vi "Regex Submatch Array.vi"(5 "multiline? (F)":bool, 6 "Submatches? (T)":bool=TRUE, 7 "ignore case? (F)":bool, 8 "error in (no error)":errorcluster, 9 "offset (0)":i32, 10 "regular expression":string, 11 "string":string) -> (0 "error out":errorcluster, 1 "offset past match":i32, 2 "after match":string, 3 "before match":string, 4 "matches":string[](array[string]))   [LabVIEW 2020, in "URI.lvlib"]
uses:
  URI.lvlib
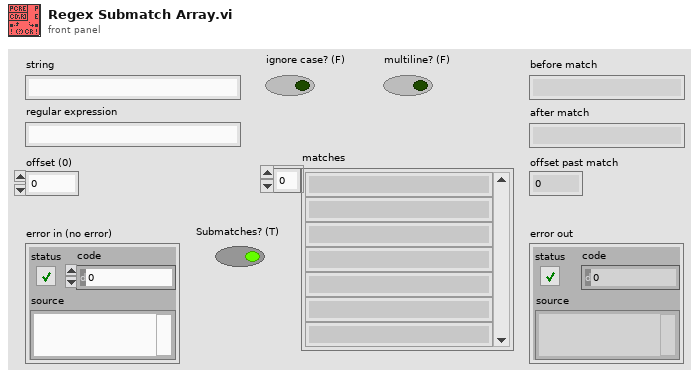
[diagram p1: front panel]
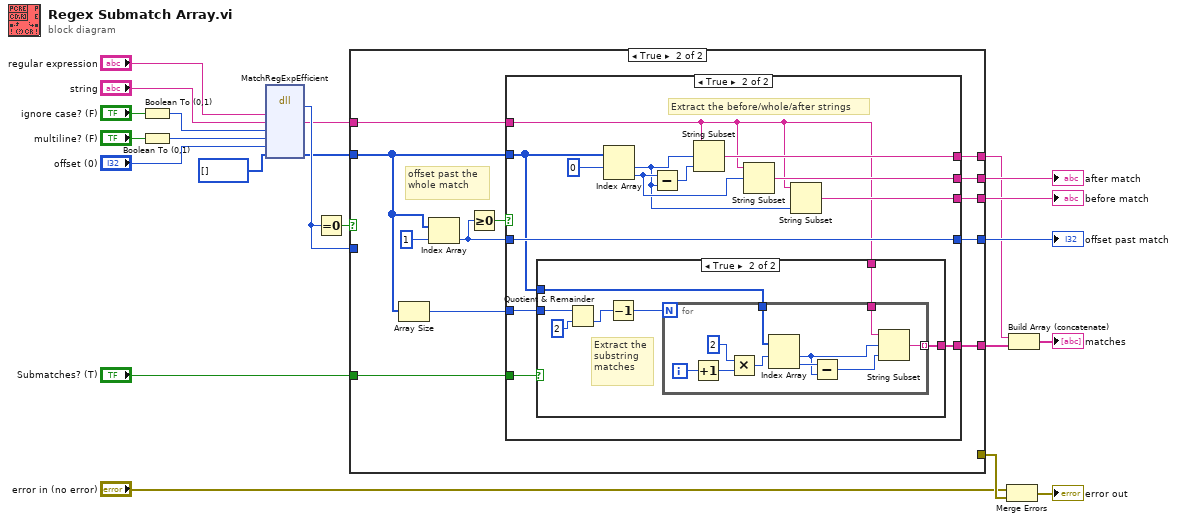
[diagram p0: block diagram]
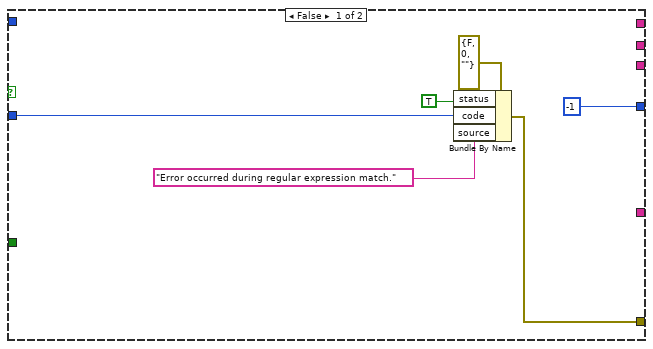
[diagram p2: hidden frame]
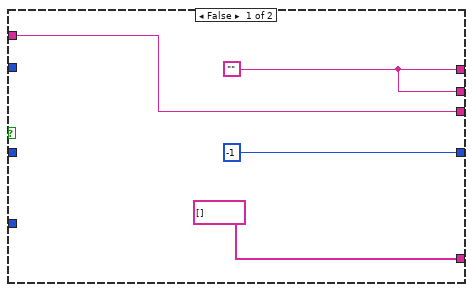
[diagram p3: hidden frame]
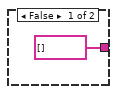
[diagram p4: hidden frame]
diagram:
  n1 = Boolean To (0,1)(Boolean="ignore case? (F)") -> (0, 1=w7:i16)
  n2 = Boolean To (0,1)(Boolean="multiline? (F)") -> (0, 1=w8:i16)
  n3 = dll-call lib="LabVIEW" fn="MatchRegExpEfficient"("regexp"="regular expression", "subject"="string", "noCase"=w7, "multiline"=w8, "offsetIn"="offset (0)", "offsetsOut"=i32[] []) -> ("return type"=w5:i32, "subject"=w3:string, "offsetsOut"=w4:i32[])  [unwired: 7 in, 2 out]
  n4 = Equal To 0?(x=w5) -> (x = 0?=w6:bool)
  n5 = case shown="True" w6 {
    tunnel: w5 -> [w24 _]
    tunnel: [w25 _] -> w17
    tunnel: w4 -> [_ w37]
    tunnel: w3 -> [_ w35]
    tunnel: [_ w34] -> w11
    tunnel: [_ w33] -> w16
    tunnel: [_ w32] -> w15
    tunnel: [-1 w31] -> w14
    tunnel: [_ w30] -> w13
    tunnel: "Submatches? (T)" -> [_ w29]
    frame False {
      n6 = Bundle By Name(cluster=errorcluster {"status"=FALSE, "code"=0, "source"=""} ("error in (no error)"), "status"=TRUE, "code"=w24, "source"="Error occurred during regular expression match.") -> (w25:errorcluster)
    }
    frame True {
      # "offset past the whole match"
      n7 = Array Size(array=w37) -> (size(s)=w39:i32)
      n8 = Index Array(array=w37, index=1) -> (element=w38:i32)
      n9 = Greater Or Equal To 0?(x=w38) -> (x >= 0?=w36:bool)
      n10 = case shown="True" w36 {
        tunnel: [string[] [] w57] -> w30
        tunnel: w35 -> [w41 w47]
        tunnel: [w42 w54] -> w34
        tunnel: w37 -> [_ w52]
        tunnel: w39 -> [_ w46]
        tunnel: [-1 w53] -> w31
        tunnel: w38 -> [_ w53]
        tunnel: [w42 w49] -> w33
        tunnel: [w41 w48] -> w32
        tunnel: w29 -> [_ w45]
        frame False {
          w42 = ""
        }
        frame True {
          # "Extract the before/whole/after strings"
          n11 = case shown="True" w45 {
            tunnel: [string[] [] w65] -> w57
            tunnel: w52 -> [_ w64]
            tunnel: w47 -> [_ w63]
            tunnel: w46 -> [_ w62]
            frame False {
            }
            frame True {
              # "Extract the substring matches"
              n12 = Quotient & Remainder(x=w62, y=2) -> (floor(x/y)=w60:i32)  [unwired: 1 out]
              n13 = Decrement(x=w60) -> (x-1=w59:i32)
              n14 = for {
                N: w59 -> [_]
                tunnel: w64 -> [w69]
                tunnel: w63 -> [w70]
                tunnel: [w66] -> w65 mode=indexing
                i -> [w67]
                n15 = Increment(x=w67) -> (x+1=w75:i32)
                n16 = Multiply(x=2, y=w75) -> (x*y=w68:i32)
                n17 = Index Array(array=w69, index #1=w68) -> (element #1=w71:i32, element #2=w72:i32)  [unwired: 1 in]
                n18 = Subtract(x=w72, y=w71) -> (x-y=w73:i32)
                n19 = String Subset(string=w70, offset (0)=w71, length (rest)=w73) -> (substring=w66:string)
              }
            }
          }
          n20 = Index Array(array=w52, index #1=0 ("index")) -> (element #1=w50:i32, element #2=w51:i32)  [unwired: 1 in]
          n21 = Subtract(x=w51, y=w50) -> (x-y=w55:i32)
          n22 = String Subset(string=w47, offset (0)=w50, length (rest)=w55) -> (substring=w54:string)
          n23 = String Subset(string=w47, offset (0)=w51) -> (substring=w49:string)  [unwired: 1 in]
          n24 = String Subset(string=w47, length (rest)=w50) -> (substring=w48:string)  [unwired: 1 in]
        }
      }
    }
  }
  "before match" <- w15
  "after match" <- w16
  "offset past match" <- w14
  n25 = Merge Errors("error in (no error)", w17) -> (→"error out":errorcluster)
  n26 = Build Array (concatenate)(w11, w13) -> (→"matches":string[])
